vi "XY Graph Save Selected Plots Event.vi"(6 "Delimiter (TAB)":string="\t", 7 "X Axis Option (Dialog)":T1(ring), 8 "Error In":errorcluster, 9 "Save All Plots? (T)":bool=TRUE, 10 "File Path in":path, 11 "XYGraph Ref":T2) -> (0 "Error Out":errorcluster, 1 "Message":string, 2 "File Path out":path, 3 "Saved Plot Names":string[](array[string]), 4 "Saved Plot Indices":i32[](array[numeric]), 5 "Graph Captiom":string)   [LabVIEW 2019, in "XY Graph Add-Ons.lvlib"]
uses:
  XY Graph Add-Ons.lvlib
  XY Graph Refnum.ctl
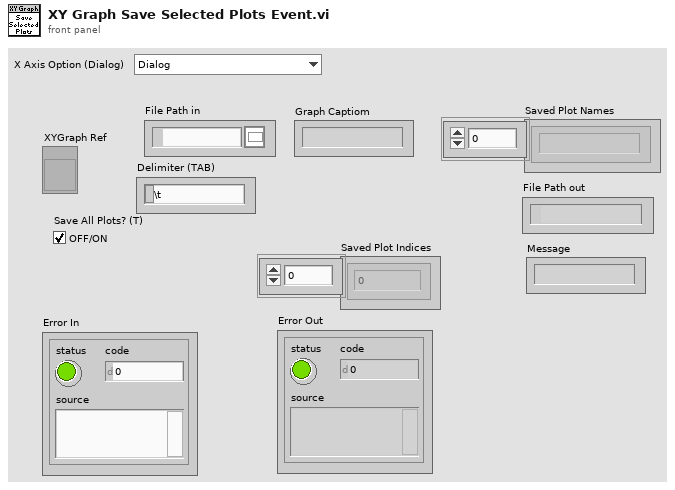
[diagram p1: front panel]
types:
  T1 = enum16{"Dialog", "Save Single X Axis if Common", "Save X Axis for each Plot"}
  T2 = typedef "XY Graph Add-Ons.lvlib/XY Graph Refnum.ctl" = refnum<vi>
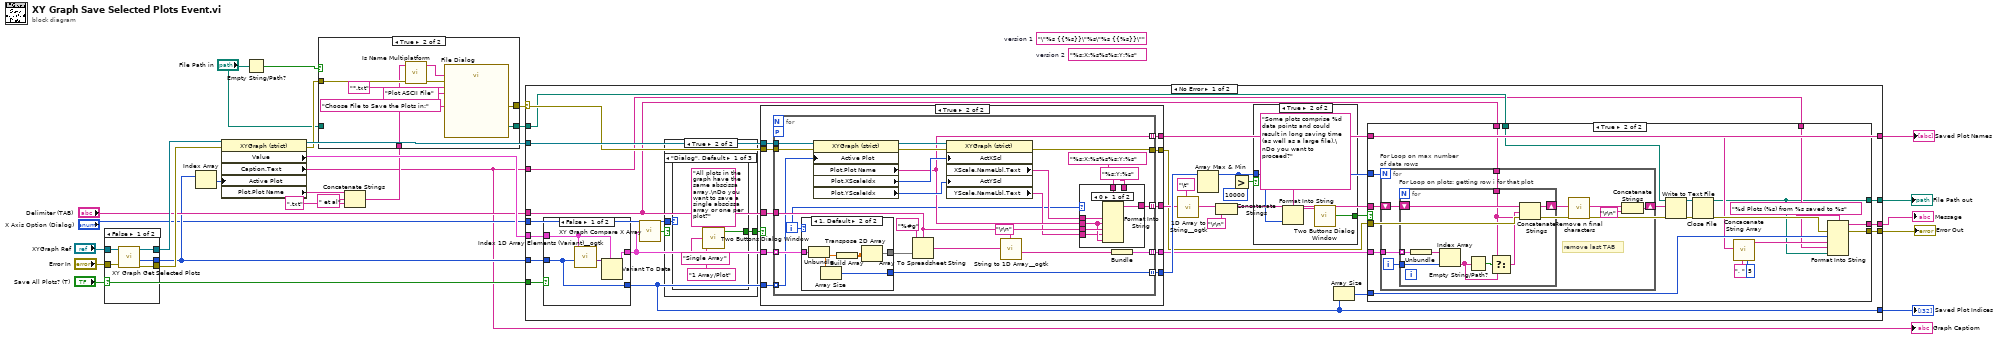
[diagram p0: block diagram]
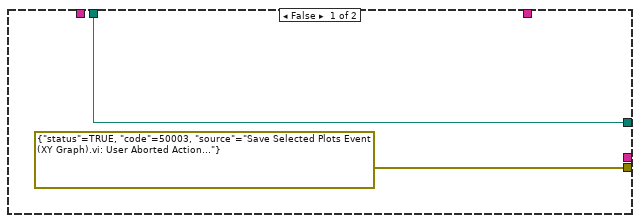
[diagram p4: hidden frame]
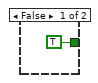
[diagram p5: hidden frame]
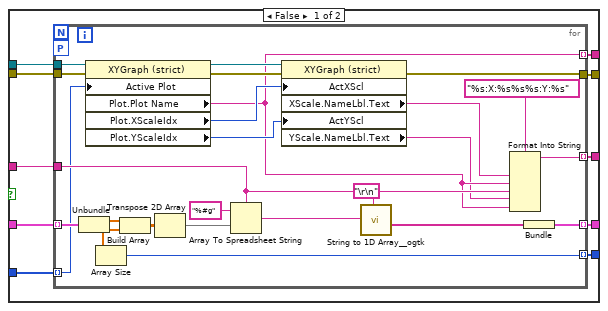
[diagram p6: hidden frame]
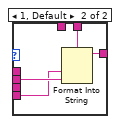
[diagram p7: hidden frame]
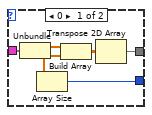
[diagram p8: hidden frame]
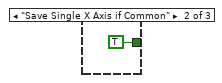
[diagram p10: hidden frame]
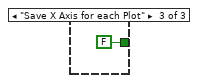
[diagram p11: hidden frame]
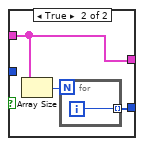
[diagram p12: hidden frame]
diagram:
  (unwired) "%s:X:%s%s%s:Y:%s"  # version 2
  (unwired) "\"%s {{%s}}\"%s\"%s {{%s}}\""  # version 1
  n1 = case shown="False" "Save All Plots? (T)" {
    tunnel: "XYGraph Ref" -> [w31 w33]
    tunnel: "Error In" -> [w30 w32]
    tunnel: [w29 w33] -> w24
    tunnel: [w28 _] -> w12
    tunnel: [w27 w32] -> w19
    frame False {
      n2 = call "XY Graph Get Selected Plots.vi"("error in (no error)"=w30, "XYGraph in"=w31) -> ("error out"=w27:errorcluster, "Selected Plots"=w28:i32[], "XYGraph out"=w29:T2)  [unwired: 5 in, 2 out]
    }
    frame True {
    }
  }
  n3 = Index Array(array=w12) -> (element=w11:i32)  [unwired: 1 in]
  n4 = property class="XYGraph (strict)"(reference=w24, error in=w19, "Active Plot"=w11) -> (reference out=w22:T2, error out=w7:errorcluster, "Value"=w23:cluster{"X Array":dbl[], "Y Array":dbl[]}[], "Caption.Text"=w1:string, "Plot.Plot Name"=w10:string)
  "Graph Captiom" <- w1
  n5 = Empty String/Path?(string/path="File Path in") -> (empty?=w5:bool)
  n6 = Concatenate Strings(w10, " et al" ("string"), ".txt" ("string")) -> (w6:string)
  n7 = case shown="True" w5 {
    tunnel: [w34 w41] -> w18
    tunnel: [w35 w40] -> w17
    tunnel: w7 -> [w34 w39]
    tunnel: w6 -> [_ w36]
    tunnel: "File Path in" -> [w35 _]
    frame False {
    }
    frame True {
      n8 = call <vilib>:"Is Name Multiplatform.vi"("error in (no error)"=w39, "filename"=w36) -> ("error out"=w38:errorcluster, "suggested filename"=w37:string)  [unwired: 5 in, 3 out]
      n9 = call "File Dialog"("prompt"="Choose File to Save the Plots in:", "default name"=w37, "error in"=w38, "pattern (all files)"="*.txt", "pattern label"="Plot ASCII File") -> ("selected path"=w40:path, "error out"=w41:errorcluster)  [unwired: 7 in, 2 out]
    }
  }
  n10 = case shown="No Error" w18 {
    selector: w18 -> [w70 w226]
    tunnel: w23 -> [w74 _]
    tunnel: w22 -> [w73 _]
    tunnel: [w46 _] -> w21
    tunnel: [w51 w226] -> w20
    tunnel: w12 -> [w63 _]
    tunnel: w17 -> [w52 _]
    tunnel: [w50 _] -> w16
    tunnel: "Save All Plots? (T)" -> [w64 _]
    tunnel: [w49 _] -> w14
    tunnel: "Delimiter (TAB)" -> [w62 _]
    tunnel: "X Axis Option (Dialog)" -> [w58 _]
    tunnel: [w47 _] -> w2
    tunnel: w1 -> [w45 _]
    frame No Error {
      n11 = case shown="False" w64 {
        tunnel: w74 -> [w220 w224]
        tunnel: [w219 w224] -> w61
        tunnel: w63 -> [w218 _]
        tunnel: [w218 w222] -> w49
        frame False {
          n12 = call <userlib>:"Index 1D Array Elements (Variant)__ogtk.vi"("indices"=w218, "array"=w220) -> ("elements"=w221:variant[])  [unwired: 9 in]
          n13 = Variant To Data(type=w220, Variant=w221) -> (data=w219:cluster{"X Array":dbl[], "Y Array":dbl[]}[])  [unwired: 1 in, 1 out]
        }
        frame True {
          n14 = Array Size(array=w224) -> (size(s)=w223:i32)
          n15 = for {
            N: w223 -> [_]
            tunnel: [w225] -> w222 mode=indexing
            i -> [w225]
          }
        }
      }
      n16 = call "XY Graph Compare X Array.vi"("Plot Array"=w61) -> ("Same [X]?"=w60:bool)  [unwired: 8 in]
      n17 = case shown="True" w60 {
        selector: w60 -> [w209 _]
        tunnel: [w209 w211] -> w59
        tunnel: w58 -> [_ w210]
        frame False {
        }
        frame True {
          n18 = case shown="\"Dialog\", Default" w210 {
            tunnel: [w212 TRUE ("T button?") FALSE ("T button?")] -> w211
            frame "Dialog", Default {
              n19 = call "Two Buttons Dialog Window.vi"("Cancel Button Text"="1 Array/Plot" ("F button name (\"Cancel\")"), "OK Button Text"="Single Array" ("T button name (\"OK\")"), "Message"="All plots in the graph have the same abscissa array.\nDo you want to save a single abscissa array or one per plot?" ("message")) -> ("OK?"=w212:bool)
            }
            frame "Save Single X Axis if Common" {
            }
            frame "Save X Axis for each Plot" {
            }
          }
        }
      }
      n20 = case shown="True" w59 {
        tunnel: w73 -> [w128 w163]
        tunnel: [w127 w162] -> w46
        tunnel: [w126 w161] -> w72
        tunnel: [w125 w160] -> w71
        tunnel: w70 -> [w124 w159]
        tunnel: [w123 w158] -> w69
        tunnel: [w122 w157] -> w53
        tunnel: w62 -> [w121 w156]
        tunnel: w49 -> [w120 w155]
        tunnel: w61 -> [w119 w154]
        frame False {
          n21 = for {
            tunnel: w119 -> [w153] mode=indexing
            tunnel: w128 -> [w152]
            tunnel: [w132] -> w127 mode=indexing
            tunnel: w124 -> [w151]
            tunnel: [w144] -> w122
            tunnel: [w134] -> w125 mode=indexing
            tunnel: [w138] -> w126 mode=indexing
            tunnel: [w140] -> w123 mode=indexing
            workers-P: _ -> [_]
            tunnel: w121 -> [w133]
            tunnel: w120 -> [w129] mode=indexing
            n22 = Unbundle(w153) -> ("X Array"=w146:dbl[], "Y Array"=w139:dbl[])
            n23 = property class="XYGraph (strict)"(reference=w152, error in=w151, "Active Plot"=w129) -> (reference out=w150:T2, error out=w145:errorcluster, "Plot.Plot Name"=w132:string, "Plot.XScaleIdx"=w143:u32, "Plot.YScaleIdx"=w142:u32)
            n24 = Array Size(array=w139) -> (size(s)=w138:i32)
            n25 = Build Array(w146, w139) -> (w149:dbl[][])
            n26 = Transpose 2D Array(2D array=w149) -> (transposed array=w148:dbl[][])
            n27 = Array To Spreadsheet String(delimiter (Tab)=w133, array=w148, 3:"%#g" ("format string")) -> (spreadsheet string=w136:string)
            n28 = property class="XYGraph (strict)"(reference=w150, error in=w145, "ActXScl"=w143, "ActYScl"=w142) -> (error out=w144:errorcluster, "XScale.NameLbl.Text"=w131:string, "YScale.NameLbl.Text"=w130:string)  [unwired: 1 out]
            n29 = call <userlib>:"String to 1D Array__ogtk.vi"("delimiter (Tab)"="\r\n", "string"=w136) -> ("Array of Strings"=w135:string[])  [unwired: 9 in]
            n30 = Format Into String(format string="%s:X:%s%s%s:Y:%s", w131, w132, w133, w130, w132) -> (resulting string=w140:string)  [unwired: 2 in, 1 out]
            n31 = Bundle("Array of Strings"=w135) -> (w134:cluster{"Array of Strings":string[]})  [unwired: 1 in]
          }
        }
        frame True {
          n32 = for {
            tunnel: w154 -> [w187] mode=indexing
            tunnel: w163 -> [w186]
            tunnel: [w169] -> w162 mode=indexing
            tunnel: w159 -> [w185]
            tunnel: [w180] -> w157
            tunnel: [w171] -> w160 mode=indexing
            tunnel: [w175] -> w161 mode=indexing
            tunnel: [w176] -> w158 mode=indexing
            workers-P: _ -> [_]
            tunnel: w156 -> [w170]
            tunnel: w155 -> [w166] mode=indexing
            i -> [w165]
            n33 = case shown="1, Default" w165 {
              tunnel: w187 -> [w203 w208]
              tunnel: [w201 w206] -> w183
              tunnel: [w198 w204] -> w175
              frame 0 {
                n34 = Unbundle(w203) -> ("X Array"=w200:dbl[], "Y Array"=w199:dbl[])
                n35 = Array Size(array=w199) -> (size(s)=w198:i32)
                n36 = Build Array(w200, w199) -> (w202:dbl[][])
                n37 = Transpose 2D Array(2D array=w202) -> (transposed array=w201:dbl[][])
              }
              frame 1, Default {
                n38 = Unbundle(w208) -> ("Y Array"=w205:dbl[])  [unwired: 1 out]
                n39 = Array Size(array=w205) -> (size(s)=w204:i32)
                n40 = Build Array(w205) -> (w207:dbl[][])
                n41 = Transpose 2D Array(2D array=w207) -> (transposed array=w206:dbl[][])
              }
            }
            n42 = property class="XYGraph (strict)"(reference=w186, error in=w185, "Active Plot"=w166) -> (reference out=w184:T2, error out=w181:errorcluster, "Plot.Plot Name"=w169:string, "Plot.XScaleIdx"=w179:u32, "Plot.YScaleIdx"=w178:u32)
            n43 = Array To Spreadsheet String(delimiter (Tab)=w170, array=w183, 3:"%#g" ("format string")) -> (spreadsheet string=w173:string)
            n44 = property class="XYGraph (strict)"(reference=w184, error in=w181, "ActXScl"=w179, "ActYScl"=w178) -> (error out=w180:errorcluster, "XScale.NameLbl.Text"=w168:string, "YScale.NameLbl.Text"=w167:string)  [unwired: 1 out]
            n45 = call <userlib>:"String to 1D Array__ogtk.vi"("delimiter (Tab)"="\r\n", "string"=w173) -> ("Array of Strings"=w172:string[])  [unwired: 9 in]
            n46 = case shown="0" w165 {
              tunnel: "%s:X:%s%s%s:Y:%s" ("format string") -> [w193 _]
              tunnel: [w192 w197] -> w176
              tunnel: w170 -> [w191 _]
              tunnel: w169 -> [w190 w196]
              tunnel: w168 -> [w189 _]
              tunnel: w167 -> [w188 w195]
              tunnel: "%s:Y:%s" ("format string") -> [_ w194]
              frame 0 {
                n47 = Format Into String(format string=w193, w189, w190, w191, w188, w190) -> (resulting string=w192:string)  [unwired: 2 in, 1 out]
              }
              frame 1, Default {
                n48 = Format Into String(format string=w194, w195, w196) -> (resulting string=w197:string)  [unwired: 2 in, 1 out]
              }
            }
            n49 = Bundle("Array of Strings"=w172) -> (w171:cluster{"Array of Strings":string[]})  [unwired: 1 in]
          }
        }
      }
      n50 = call <userlib>:"1D Array to String__ogtk.vi"("delimiter (Tab)"="\t", "Array of Strings"=w69) -> ("delimited string"=w67:string)  [unwired: 9 in]
      n51 = Array Max & Min(array=w72) -> (max value=w55:i32)  [unwired: 3 out]
      n52 = Concatenate Strings(w67, "\r\n") -> (w66:string)
      n53 = Greater?(x=w55, y=10000) -> (0:w56:bool)
      n54 = case shown="True" w56 {
        tunnel: [TRUE ("T button?") w116] -> w54
        tunnel: w55 -> [_ w115]
        frame False {
        }
        frame True {
          n55 = Format Into String(format string="Some plots comprise %d data points and could result in long saving time (as well as a large file).\nDo you want to proceed?", w115) -> (resulting string=w117:string)  [unwired: 2 in, 1 out]
          n56 = call "Two Buttons Dialog Window.vi"("Message"=w117) -> ("OK?"=w116:bool)  [unwired: 2 in]
        }
      }
      n57 = Array Size(array=w49) -> (size(s)=w48:i32)
      n58 = case shown="True" w54 {
        tunnel: w71 -> [_ w96]
        tunnel: w66 -> [_ w95]
        tunnel: w62 -> [_ w94]
        tunnel: w55 -> [_ w93]
        tunnel: w53 -> [_ w92]
        tunnel: w52 -> [w76 w90]
        tunnel: [errorcluster {"status"=TRUE, "code"=50003, "source"="Save Selected Plots Event (XY Graph).vi: User Aborted Action..."} ("error IO") w83] -> w51
        tunnel: [w76 w77] -> w50
        tunnel: w48 -> [_ w82]
        tunnel: [_ w80] -> w47
        tunnel: w46 -> [_ w79]
        tunnel: w45 -> [_ w78]
        frame False {
        }
        frame True {
          n59 = for "For Loop on max number of data rows" {
            N: w93 -> [_]
            tunnel: w96 -> [w104]
            shift-right: [w100] -> w91
            shift-left: w95 -> [w103]
            tunnel: w94 -> [w97]
            i -> [w102]
            # "remove last TAB"
            n60 = for "For Loop on plots: getting row i for that plot" {
              tunnel: w104 -> [w113] mode=indexing
              shift-right: [w106] -> w101
              shift-left: w103 -> [w108]
              tunnel: w102 -> [w111]
              tunnel: w97 -> [w105]
              n61 = Unbundle(w113) -> ("Array of Strings"=w112:string[])
              n62 = Index Array(array=w112, index=w111) -> (element=w109:string)
              n63 = Empty String/Path?(string/path=w109) -> (empty?=w110:bool)
              n64 = Select(t=w105, s=w110, f=w109) -> (s? t:f=w107:string)
              n65 = Concatenate Strings(w108, w107, w105) -> (w106:string)
            }
            n66 = call "Remove n final characters.vi"("String in"=w101) -> ("String out"=w98:string)  [unwired: 8 in]
            n67 = Concatenate Strings(w98, "\r\n") -> (w100:string)
          }
          n68 = Write to Text File(file (use dialog)=w90, text=w91, error in=w92) -> (refnum out=w88:refnum<file>, error out=w89:errorcluster)  [unwired: 1 in, 1 out]
          n69 = Close File(refnum=w88, error in=w89) -> (path=w77:path, error out=w84:errorcluster)
          n70 = call "Concacenate String Array.vi"("Max Number of Elements (None: -1)"=5 ("Max Number of Elements (None: 1)"), "Separator (TAB)"=", ", "String Array"=w79) -> ("Formatted String"=w85:string)  [unwired: 8 in]
          n71 = Format Into String(format string="%d Plots (%s) from %s saved to %s", error in=w84, w82, w85, w78, w77) -> (resulting string=w80:string, error out=w83:errorcluster)  [unwired: 1 in]
        }
      }
    }
    frame Error {
    }
  }
  "Error Out" <- w20
  "Saved Plot Indices" <- w14
  "Saved Plot Names" <- w21
  "File Path out" <- w16
  "Message" <- w2
